vi "Operator-Panel.vi"() -> ()   [LabVIEW 2021]
uses:
  Global-Var-OperService.vi
  Global-Var-Simulator.vi
panel:
  in  "all_alarm_delete button":bool
  in  "service_workAck_btn":bool
  in  "home_btn":bool
  out "carWash_2_alarm_ind_2":bool
  out "carWash_1_alarm_ind_2":bool
  out "service_work_finished_ind":bool
  out "service_work_started_ind":bool
  out "service_call_received_ind":bool
  out "service_call_sent_ind":bool
  in  "call_service_btn":bool
  out "carWash_2_alarm_ind":bool
  out "carWash_2_status_ind":bool
  in  "carWash_2_btn":bool
  out "carWash_1_alarm_ind":bool
  out "carWash_1_status_ind":bool
  in  "carWash_1_btn":bool
  # "Alarmy"
  # "Myjnia Południe"
  # "Myjnia Północ"
  # "Kasuj wszystkie alarmy"
  # "Serwis naprawczy"
  # "Serwisant rozpoczął\npracę"
  # "Serwisant wezwany"
  # "Serwisant odebrał\nzgłoszenie"
  # "Serwisant zakończył\npracę"
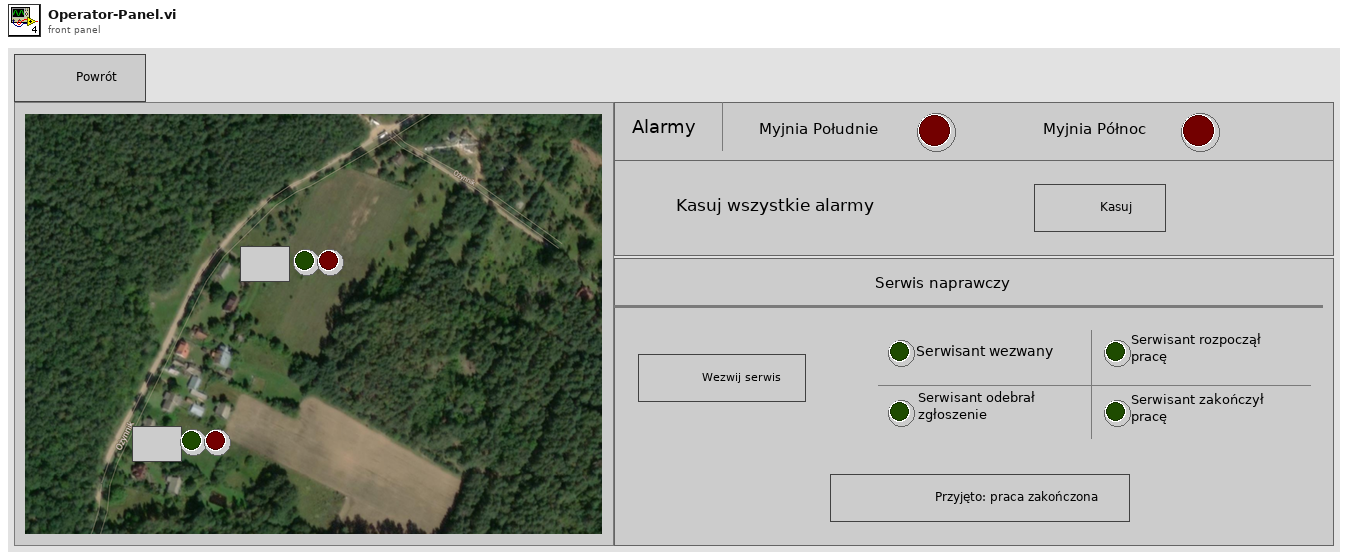
[diagram p1: front panel]
types:
  T1 = enum32{"Invalid", "Standard", "Closed", "Hidden", "Minimized", "Maximized"}
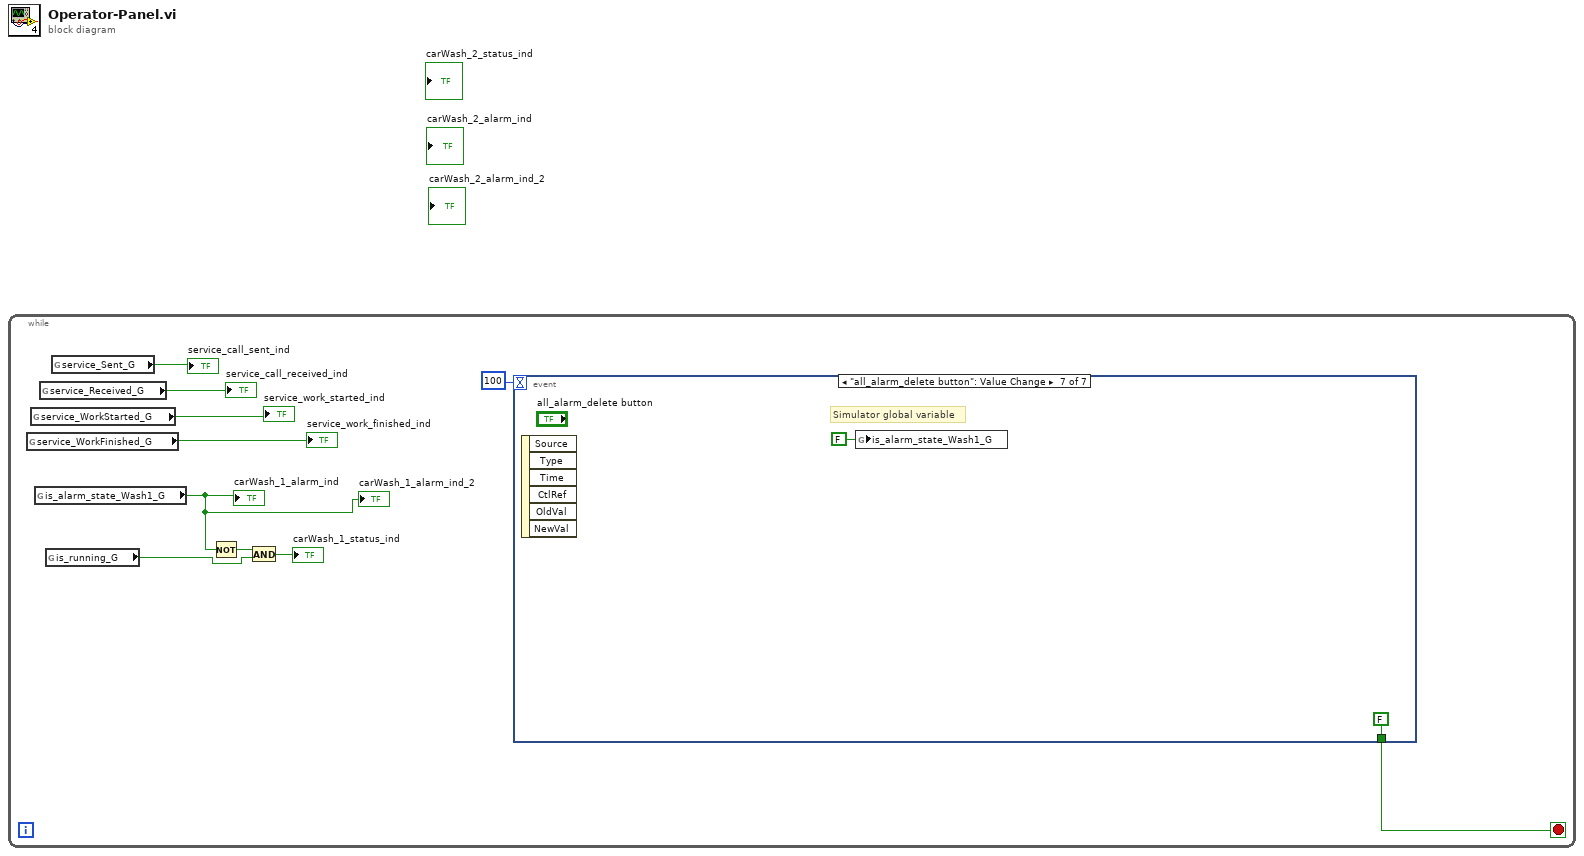
[diagram p0: block diagram]
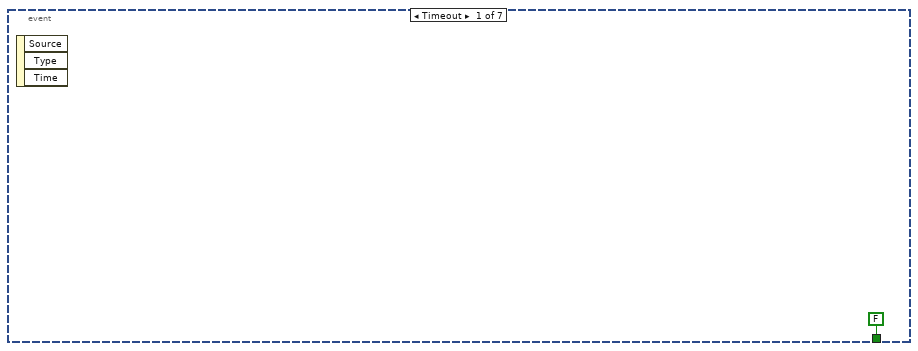
[diagram p2: hidden frame]
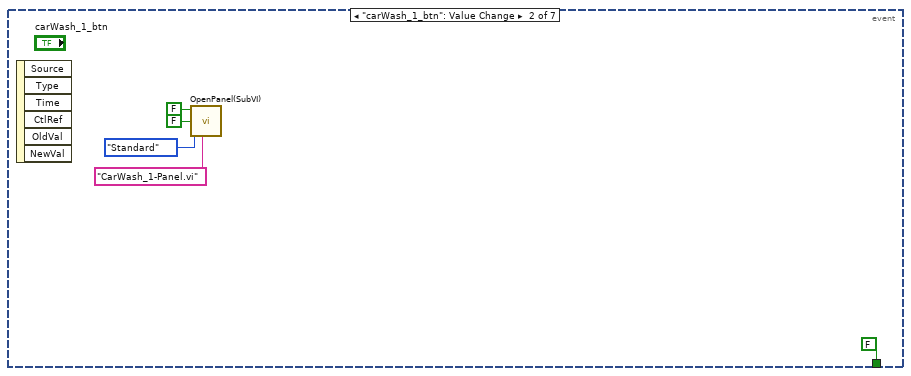
[diagram p3: hidden frame]
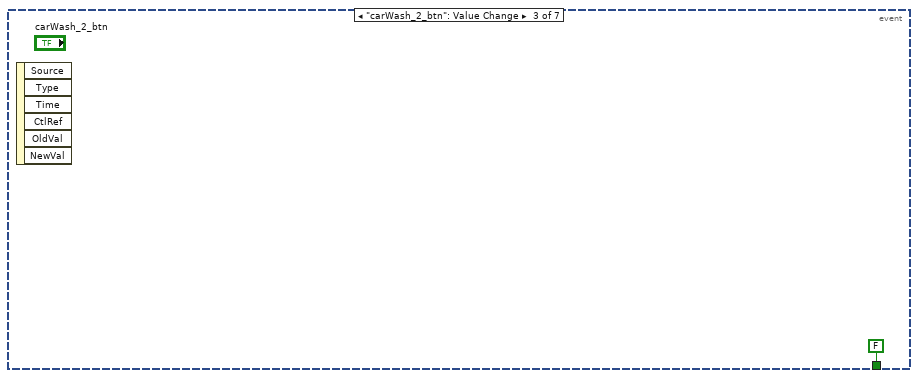
[diagram p4: hidden frame]
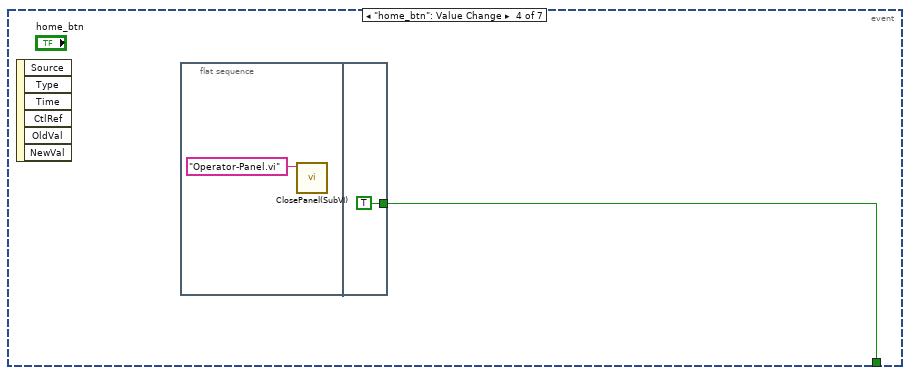
[diagram p5: hidden frame]
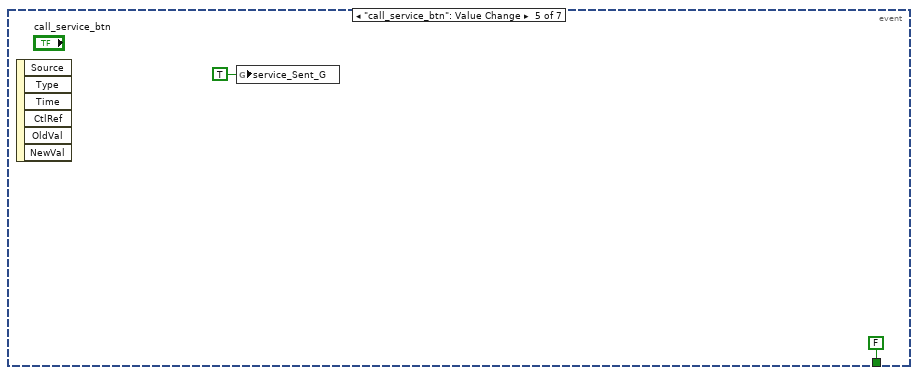
[diagram p6: hidden frame]
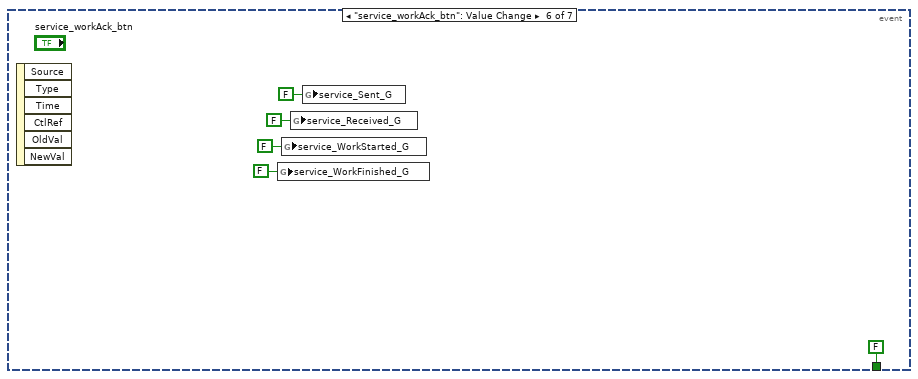
[diagram p7: hidden frame]
diagram:
  n1 = while {
    stop <- w9 stop-if-true
    n2 = global read "Global-Var-OperService.vi" "service_WorkFinished_G"() -> (→"service_work_finished_ind":bool)
    n3 = global read "Global-Var-OperService.vi" "service_WorkStarted_G"() -> (→"service_work_started_ind":bool)
    n4 = global read "Global-Var-Simulator.vi" "is_alarm_state_Wash1_G"() -> (w1:bool)
    "carWash_1_alarm_ind" <- w1
    "carWash_1_alarm_ind_2" <- w1
    n5 = global read "Global-Var-OperService.vi" "service_Received_G"() -> (→"service_call_received_ind":bool)
    n6 = global read "Global-Var-Simulator.vi" "is_running_G"() -> (w3:bool)
    n7 = global read "Global-Var-OperService.vi" "service_Sent_G"() -> (→"service_call_sent_ind":bool)
    n8 = Not(x=w1) -> (.not. x?=w4:bool)
    n9 = And(x=w4, y=w3) -> (x .and. y?=→"carWash_1_status_ind":bool)
    n10 = event shown="[6] \"all_alarm_delete button\": Value Change" {
      selector: _ -> [_ _ _ _ _ _ _]
      dyn-events: _ -> [_ _ _ _ _ _ _]
      timeout: 100 -> [_ _ _ _ _ _ _]
      tunnel: [FALSE FALSE FALSE w18 FALSE FALSE FALSE] -> w9
      event Timeout {
        n11 = event-data() -> ()  [unwired: 1 in, 3 out]
      }
      event "carWash_1_btn": Value Change {
        n12 = event-data() -> ()  [unwired: 1 in, 6 out]
        n13 = call "OpenPanel(SubVI).vi"("String"="CarWash_1-Panel.vi", "State"=T1."Standard", "Wait Until Done"=FALSE, "Auto Dispose Reference"=FALSE) -> ()  [unwired: 8 in]
      }
      event "carWash_2_btn": Value Change {
        n14 = event-data() -> ()  [unwired: 1 in, 6 out]
      }
      event "home_btn": Value Change {
        n15 = event-data() -> ()  [unwired: 1 in, 6 out]
        n16 = flat-sequence {
          tunnel: [TRUE] -> w18
          frame #0 {
            n17 = call "ClosePanel(SubVI).vi"("String"="Operator-Panel.vi") -> ()  [unwired: 11 in]
          }
          frame #1 {
          }
        }
      }
      event "call_service_btn": Value Change {
        n18 = event-data() -> ()  [unwired: 1 in, 6 out]
        n19 = global write "Global-Var-OperService.vi" "service_Sent_G"(TRUE ("service_Sent_G")) -> ()
      }
      event "service_workAck_btn": Value Change {
        n20 = event-data() -> ()  [unwired: 1 in, 6 out]
        n21 = global write "Global-Var-OperService.vi" "service_WorkFinished_G"(FALSE ("service_WorkFinished_G")) -> ()
        n22 = global write "Global-Var-OperService.vi" "service_WorkStarted_G"(FALSE ("service_WorkStarted_G")) -> ()
        n23 = global write "Global-Var-OperService.vi" "service_Received_G"(FALSE ("service_Received_G")) -> ()
        n24 = global write "Global-Var-OperService.vi" "service_Sent_G"(FALSE ("service_Sent_G")) -> ()
      }
      event "all_alarm_delete button": Value Change {
        # "Simulator global variable"
        n25 = event-data() -> ()  [unwired: 1 in, 6 out]
        n26 = global write "Global-Var-Simulator.vi" "is_alarm_state_Wash1_G"(FALSE ("is_alarm_state_Wash1_G")) -> ()
      }
    }
  }
